vi "DrawHeading.vi"(1 "(xr,yr) old":cluster{"x robot":dbl, "y robot":dbl}, 2 "Heading":dbl, 3 "2D Picture":picture) -> (0 "new picture":picture)   [LabVIEW 2012]
doc: "Draws a magenta circle at the curretn (x,y) coordinates of the Robot in the current mission definition file.\nInputs:\nPicture to draw on\nCluster X\n y coordinates of robot\nOutput:\nmodified picture"
panel:
  # "Draws a circle at the current x,y coordinates of the robot"
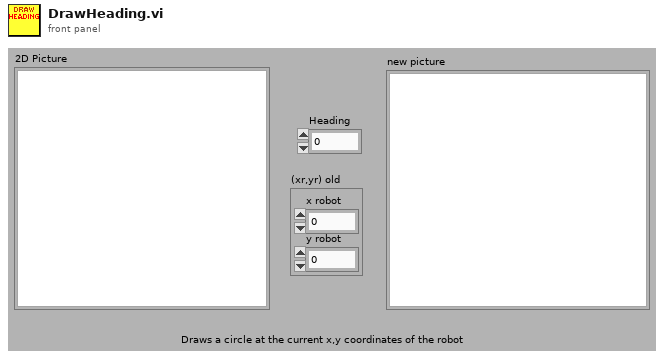
[diagram p1: front panel]
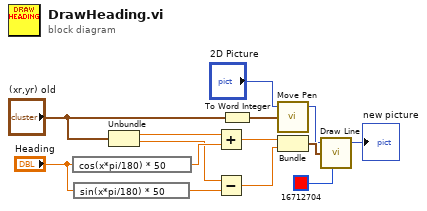
[diagram p0: block diagram]
diagram:
  n1 = expression code="cos(x*pi/180) * 50"("Heading") -> (w10:dbl)
  n2 = expression code="sin(x*pi/180) * 50"("Heading") -> (w7:dbl)
  n3 = Unbundle("(xr,yr) old") -> ("x robot"=w9:dbl, "y robot"=w8:dbl)
  n4 = Add(x=w9, y=w10) -> (x+y=w5:dbl)
  n5 = Subtract(x=w8, y=w7) -> (x-y=w6:dbl)
  n6 = To Word Integer(number="(xr,yr) old") -> (16bit integer=w14:cluster{"x robot":i16, "y robot":i16})
  n7 = call <vilib>:"Move Pen.vi"("new position"=w14, "picture"="2D Picture") -> ("new picture"=w2:picture)  [unwired: 3 in]
  n8 = Bundle(w5, w6) -> (w4:cluster{dbl, dbl})  [unwired: 1 in]
  n9 = call <vilib>:"Draw Line.vi"("picture"=w2, "end point"=w4, "color(black)"=u32 16712704) -> ("new picture"=→"new picture":picture)  [unwired: 6 in]
